vi "SetBackgroundColor.vi"(0 "reference in":refnum<class "DataGridView.lvclass">, 5 "Color":u32(colorbox), 11 "error in (no error)":errorcluster) -> (4 "reference out":refnum<class "DataGridView.lvclass">, 15 "error out":errorcluster)   [LabVIEW 2018, in "DataGridView.lvclass"]
doc: "Sets the background color of the DataGridView."
uses:
  DataGridView.lvclass
  System.Windows.Forms
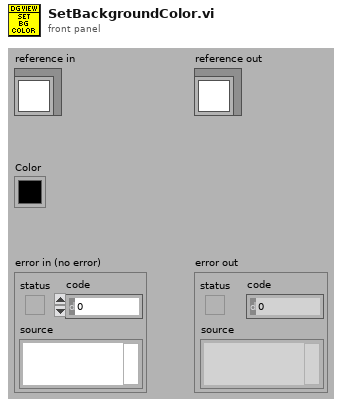
[diagram p1: front panel]
types:
  T1 = typedef "DataGridView.lvclass/ObjectAttributes.ctl" = cluster{"DataGridView":refnum<k24>, "SelectionChangedEvent":refnum<user-event>, "SelectionChanged callback ref":refnum<k27>, "LastSelectedRowIndex":i32}
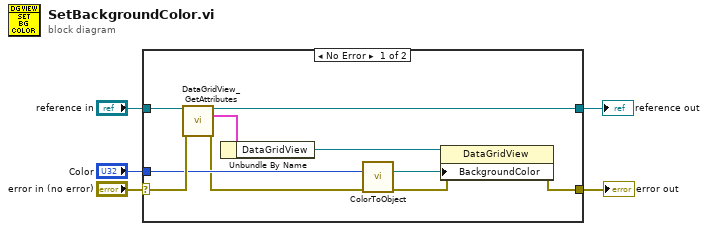
[diagram p0: block diagram]
diagram:
  n1 = case shown="No Error" "error in (no error)" {
    selector: "error in (no error)" -> [w15 w17]
    tunnel: [w8 w17] -> w4
    tunnel: [w12 w16] -> w2
    tunnel: "reference in" -> [w13 w16]
    tunnel: "Color" -> [w10 _]
    frame No Error {
      n2 = call "DataGridView_GetAttributes.vi"("reference in"=w13, "error in (no error)"=w15) -> ("reference out"=w12:refnum<class "DataGridView.lvclass">, "Data"=w14:T1, "error out"=w9:errorcluster)  [unwired: 10 in, 1 out]
      n3 = Unbundle By Name(w14) -> ("DataGridView"=w11:refnum<k24>)
      n4 = call "ColorToObject.vi"("Color"=w10, "error in (no error)"=w9) -> (".Net Color"=w6:refnum<k24>, "error out"=w7:errorcluster)  [unwired: 12 in]
      n5 = property class="DataGridView"(reference=w11, error in=w7, "BackgroundColor"=w6) -> (error out=w8:errorcluster)  [unwired: 1 out]
    }
    frame Error {
    }
  }
  "error out" <- w4
  "reference out" <- w2
